vi "Frame-Parser.vi"() -> ()   [LabVIEW 2017]
panel:
  in  "hi":u8
  out "FXP":u8
  out "(hi.lo)":u16
  in  "FXP":fxp<+,4,4>
  out "CRC OK?":bool
  out "Source MAC":u8[](array[numeric])=[0, 1, 8, 0, 6, 4] format="%02x"
  out "Destination MAC":u8[](array[numeric])=[201, 85, 8, 68, 8, 6] format="%02x"
  out "Target":cluster{"THA":u8[], "TPA":u8[]}={"THA"=[0, 0, 0, 0, 0, 0], "TPA"=[192, 168, 1, 201]} {"THA" format="%02x"}
  out "Sender":cluster{"SHA":u8[], "SPA":u8[]}={"SHA"=[0, 35, 38, 182, 175, 53], "SPA"=[192, 168, 1, 200]} {"SHA" format="%02x"}
  out "Header":T1={"HTYPE"=1, "PTYPE"=2048, "HLEN"=6, "PLEN"=4, "OPER"=1}
  out "EtherType":u16=1 format="%04x"
  out "U8 [] out":u8[](array[numeric]) format="%.0x"
  in  "Raw Data":u32[](array[numeric]) format="%.0x"
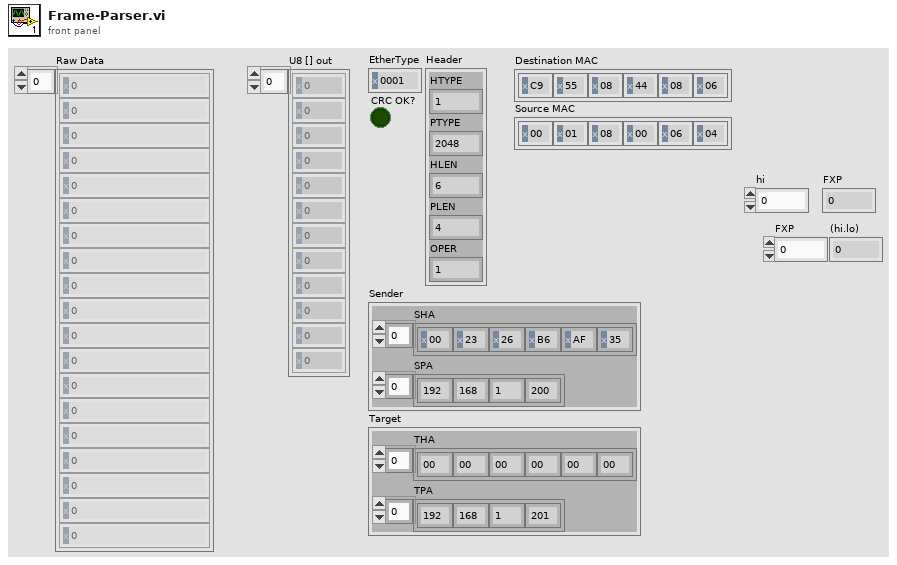
[diagram p1: front panel]
types:
  T1 = cluster{"HTYPE":u16, "PTYPE":u16, "HLEN":u8, "PLEN":u8, "OPER":u16}
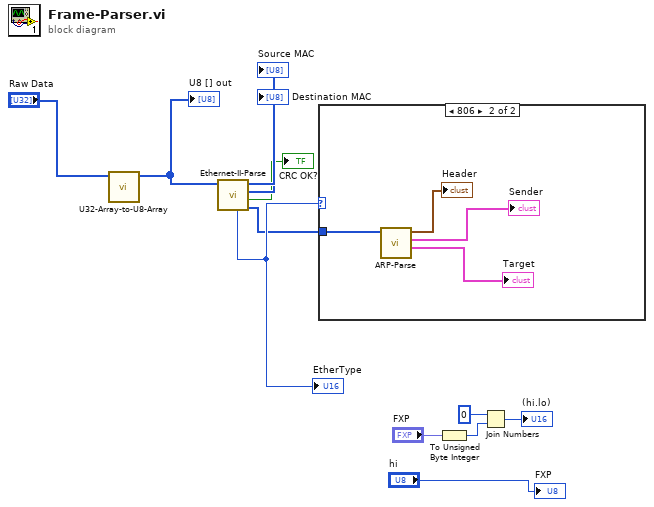
[diagram p0: block diagram]
diagram:
  n1 = call "U32-Array-to-U8-Array.vi"("U32 [] in"="Raw Data") -> ("U8 [] out"=w11:u8[])  [unwired: 10 in]
  "U8 [] out" <- w11
  n2 = call "Ethernet-II-Parse.vi"("Input Frame"=w11) -> ("Payload"=w9:u8[], "CRC OK?"=→"CRC OK?":bool, "Source MAC"=→"Source MAC":u8[], "Destination MAC"=→"Destination MAC":u8[], "EtherType"=w10:u16)  [unwired: 6 in]
  "EtherType" <- w10
  n3 = case shown="806" w10 {
    tunnel: w9 -> [_ w16]
    frame 0, Default {
    }
    frame 2054 {
      n4 = call "ARP-Parse.vi"("Frame (in)"=w16) -> ("Target"=→"Target":cluster{"THA":u8[], "TPA":u8[]}, "Sender"=→"Sender":cluster{"SHA":u8[], "SPA":u8[]}, "Header"=→"Header":T1)  [unwired: 8 in]
    }
  }
  n5 = To Unsigned Byte Integer(number="FXP") -> (unsigned 8bit integer=w1:u8)
  n6 = Join Numbers(hi=u8 0, lo=w1) -> ((hi.lo)=→"(hi.lo)":u16)
  "FXP" <- "hi"
